vi "NAND.vi"(1 "b":bool, 2 "a":bool) -> (0 "x":bool)   [LabVIEW 2012]
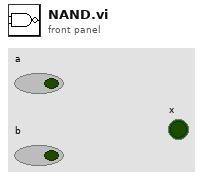
[diagram p1: front panel]
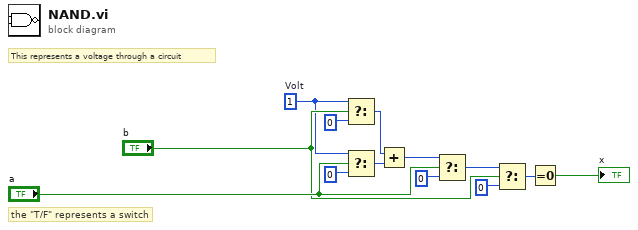
[diagram p0: block diagram]
diagram:
  w9 = 1  # Volt
  # "This represents a voltage through a circuit"
  # "the \"T/F\" represents a switch"
  n1 = Select(t=w9, s="b", f=0) -> (s? t:f=w5:i32)
  n2 = Select(t=w9, s="a", f=0) -> (s? t:f=w6:i32)
  n3 = Add(x=w5, y=w6) -> (x+y=w4:i32)
  n4 = Select(t=w4, s="a", f=0) -> (s? t:f=w10:i32)
  n5 = Select(t=w10, s="b", f=0) -> (s? t:f=w1:i32)
  n6 = Equal To 0?(x=w1) -> (x = 0?=→"x":bool)
